vi "6-5.vi"() -> ()   [LabVIEW 2017]
panel:
  in  "access (0:read/write)":enum16{"read/write", "read-only", "write-only"}(ring)
  in  "operation (0:open)":T1(ring)
  in  "file path (use dialog)":path
  out "Waveform Chart":dbl(graph)
  in  "Stop Button":bool
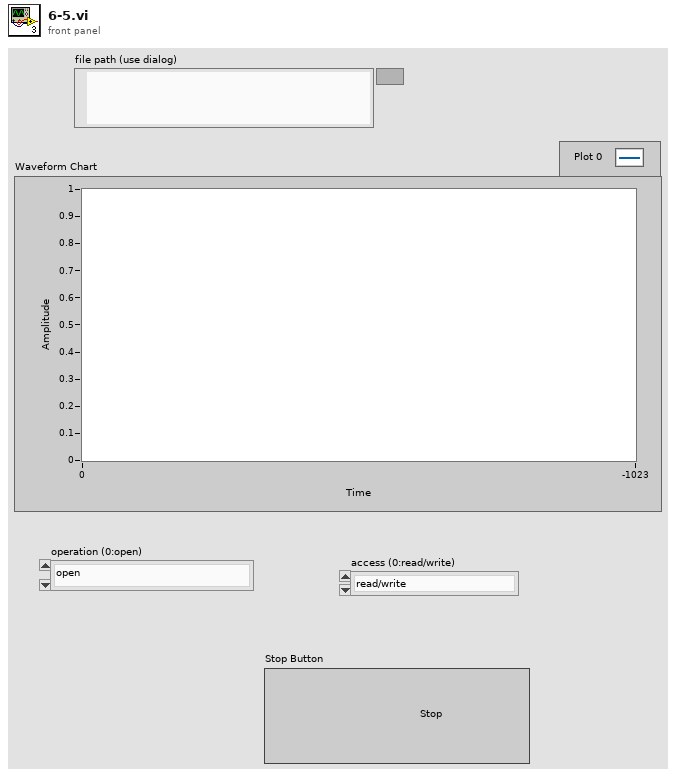
[diagram p1: front panel]
types:
  T1 = enum16{"open", "replace", "create", "open or create", "replace or create", "replace or create with confirmation"}
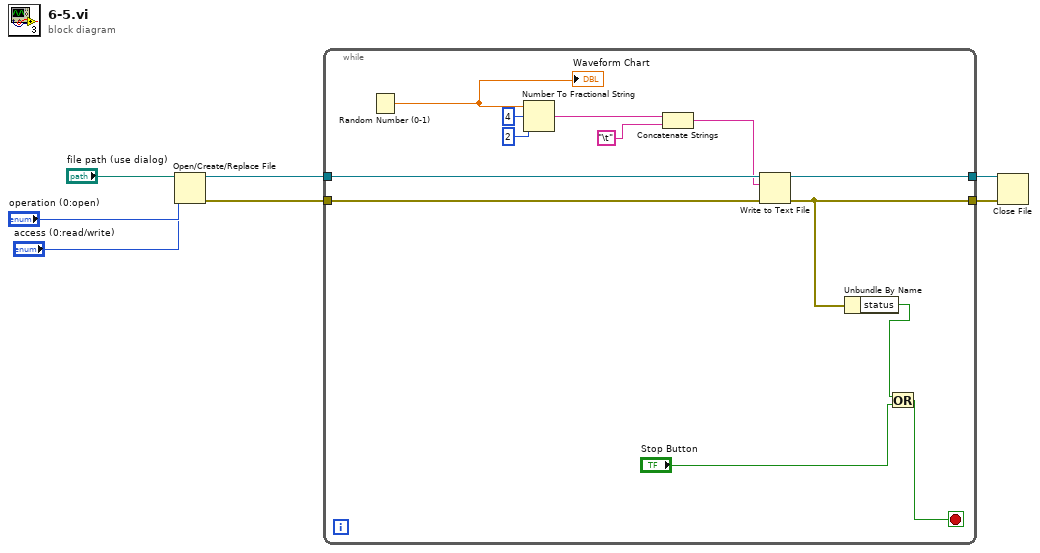
[diagram p0: block diagram]
diagram:
  n1 = Open/Create/Replace File(file path (use dialog)="file path (use dialog)", operation (0:open)="operation (0:open)", access (0:read/write)="access (0:read/write)") -> (refnum out=w7:refnum<file>, error out=w6:errorcluster)  [unwired: 3 in, 1 out]
  n2 = while {
    tunnel: w7 -> [w17]
    tunnel: w6 -> [w18]
    tunnel: [w9] -> w4
    tunnel: [w10] -> w5
    stop <- w20 stop-if-true
    n3 = Random Number (0-1)() -> (number: 0 to 1=w14:dbl)
    "Waveform Chart" <- w14
    n4 = Number To Fractional String(number=w14, width (-)=i16 4, precision (6)=i16 2) -> (F-format string=w13:string)  [unwired: 1 in]
    n5 = Concatenate Strings(w13, "\t") -> (w11:string)
    n6 = Write to Text File(file (use dialog)=w17, text=w11, error in=w18) -> (refnum out=w10:refnum<file>, error out=w9:errorcluster)  [unwired: 1 in, 1 out]
    n7 = Unbundle By Name(w9) -> ("status"=w8:bool)
    n8 = Or(x=w8, y="Stop Button") -> (x .or. y?=w20:bool)
  }
  n9 = Close File(refnum=w5, error in=w4) -> ()  [unwired: 2 out]
